vi "GetMinSampleRate.vi"(8 "error in (no error)":errorcluster, 9 "PSU Update":bool, 10 "stop":bool, 11 "min sample rate":dbl) -> (0 "error out":errorcluster, 3 "min sample rate":dbl)   [LabVIEW 2013]
uses:
  Private/Unused/PSU updated.vi
  <vilib>/addons/database/Connection.llb/Conn Execute.vi
  <vilib>/addons/database/Recordset.llb/Rec Fetch Recordset Data (R).vi
  <vilib>/addons/database/Recordset.llb/Rec Destroy - Connection.vi
  <vilib>/addons/database/_DB Variant To Data/Database Variant To Data.xnode
  <vilib>/addons/database/NI_Database_API.lvlib
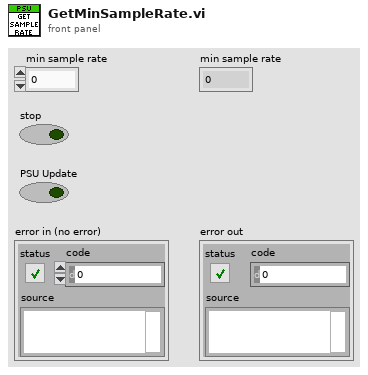
[diagram p1: front panel]
types:
  T1 = typedef "NI_Database_API.lvlib/Conn ObjectReference.ctl" = refnum<k1>
  T2 = typedef "NI_Database_API.lvlib/Rec ObjectReference.ctl" = refnum<k1>
  T3 = cluster{"Integer Timestamp":dbl, "Max Velocity":dbl, "Min Velocity":dbl}
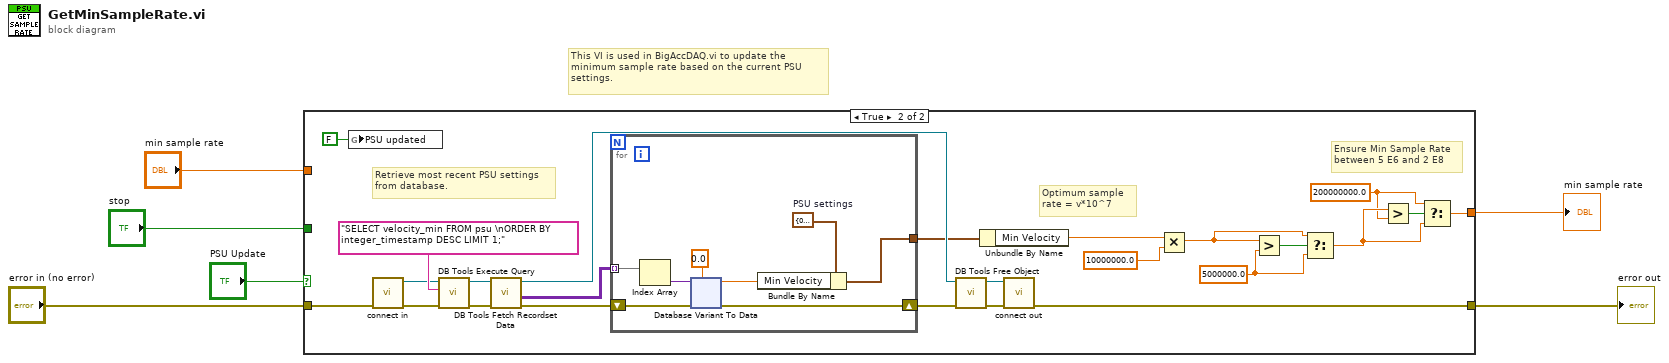
[diagram p0: block diagram]
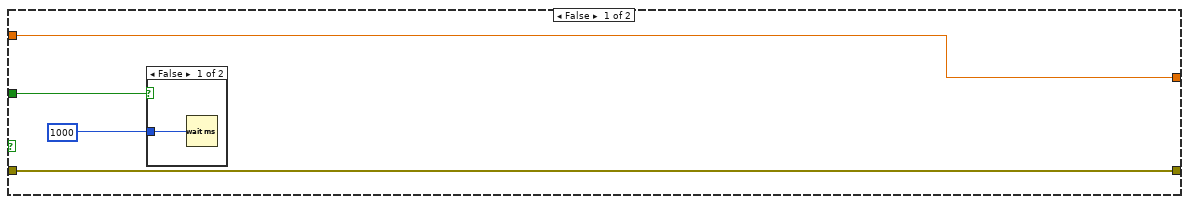
[diagram p2: hidden frame]
diagram:
  # "This VI is used in BigAccDAQ.vi to update the \nminimum sample rate based on the current PSU \nsettings."
  n1 = case shown="True" "PSU Update" {
    tunnel: "error in (no error)" -> [w10 w15]
    tunnel: [w10 w35] -> w2
    tunnel: "stop" -> [w9 _]
    tunnel: [w7 w12] -> w5
    tunnel: "min sample rate" -> [w7 _]
    frame False {
      n2 = case shown="False" w9 {
        tunnel: 1000 -> [w11 _]
        frame False {
          n3 = Wait (ms)(milliseconds to wait=w11) -> ()  [unwired: 1 out]
        }
        frame True {
        }
      }
    }
    frame True {
      w16 = 200000000.0 ("y")
      w14 = 5000000.0 ("y")
      # "Optimum sample\nrate = v*10^7"
      # "Ensure Min Sample Rate\nbetween 5 E6 and 2 E8"
      # "Retrieve most recent PSU settings \nfrom database."
      n4 = global write "PSU updated.vi" "PSU updated"(FALSE ("PSU updated")) -> ()
      n5 = call "connect in.vi"("error in (no error)"=w15) -> ("error out"=w26:errorcluster, "Database Connection"=w25:T1)  [unwired: 6 in, 1 out]
      n6 = call-poly <vilib>:"DB Tools Execute Query.vi"("error in (no error)"=w26, "SQL query"="SELECT velocity_min FROM psu \nORDER BY integer_timestamp DESC LIMIT 1;", "connection reference"=w25) -> ("error out"=w28:errorcluster, "recordset reference"=w27:T2)  [unwired: 5 in]
      n7 = call-poly <vilib>:"DB Tools Fetch Recordset Data.vi"("error in (no error)"=w28, "recordset reference"=w27) -> ("error out"=w34:errorcluster, "recordset data"=w33:variant[][], "recordset reference out"=w29:T2)  [unwired: 3 in]
      n8 = for {
        tunnel: w33 -> [w43] mode=indexing
        shift-right: [w37] -> w23
        shift-left: w34 -> [w41]
        tunnel: [w36] -> w24
        w40 = T3 {"Integer Timestamp"=0.0, "Max Velocity"=0.0, "Min Velocity"=0.0}  # PSU settings
        n9 = Index Array(array=w43) -> (element=w42:variant)  [unwired: 1 in]
        n10 = xnode "Database Variant To Data"("database variant"=w42, "error in (no error)"=w41, "type"=0.0) -> ("data"=w39:dbl, "error out"=w37:errorcluster)
        n11 = Bundle By Name(cluster=w40, "Min Velocity"=w39) -> (w36:T3)
      }
      n12 = call-poly <vilib>:"DB Tools Free Object.vi"("error in (no error)"=w23, "recordset reference"=w29) -> ("error out"=w30:errorcluster, "connection reference"=w31:T1)  [unwired: 8 in]
      n13 = Unbundle By Name(w24) -> ("Min Velocity"=w21:dbl)
      n14 = call "connect out.vi"("error in (no error)"=w30, "connection reference"=w31) -> ("error out"=w35:errorcluster)  [unwired: 9 in]
      n15 = Multiply(x=w21, y=10000000.0) -> (x*y=w13:dbl)
      n16 = Greater?(x=w13, y=w14) -> (0:w19:bool)
      n17 = Select(t=w13, s=w19, f=w14) -> (s? t:f=w18:dbl)
      n18 = Greater?(x=w18, y=w16) -> (0:w17:bool)
      n19 = Select(t=w16, s=w17, f=w18) -> (s? t:f=w12:dbl)
    }
  }
  "min sample rate" <- w5
  "error out" <- w2
